vi "CH1_Rx_TCPIP.vi"() -> ()   [LabVIEW 2018]
uses:
  RxTx/RxTx.lvclass
  TCPIP/TCPIP.lvclass
  TCPIP/TCPIP.lvclass/TCPIP.ctl
panel:
  in  "TCPIP.lvclass":refnum<class "TCPIP.lvclass">
  in  "remote port":u16=2000
  in  "IP":string="200.131.64.48"
  in  "RxTx.lvclass":refnum<class "RxTx.lvclass">
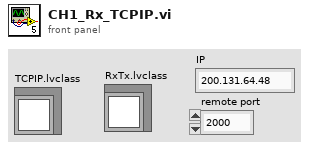
[diagram p1: front panel]
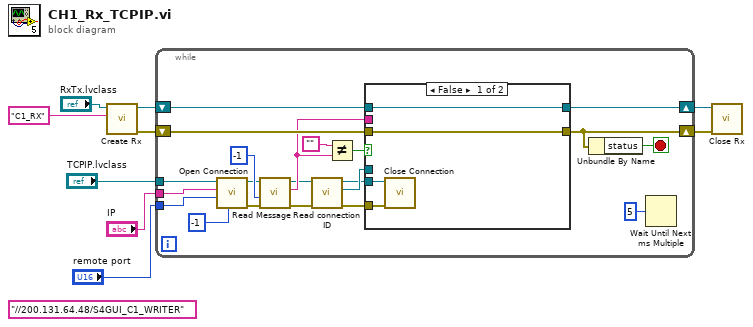
[diagram p0: block diagram]
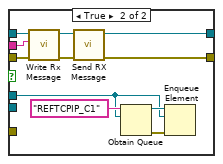
[diagram p2: hidden frame]
diagram:
  (unwired) "//200.131.64.48/S4GUI_C1_WRITER" ("witer name")
  n1 = call "Create Rx.vi"("Reader Name"="C1_RX", "RxTx in"="RxTx.lvclass") -> ("error out"=w6:errorcluster, "RxTx out"=w7:refnum<class "RxTx.lvclass">)  [unwired: 8 in]
  n2 = while {
    shift-right: [w27] -> w4
    shift-left: w6 -> [w30]
    shift-right: [w28] -> w5
    shift-left: w7 -> [w29]
    tunnel: "IP" -> [w23]
    tunnel: "remote port" -> [w22]
    tunnel: "TCPIP.lvclass" -> [w13]
    stop <- w24 stop-if-true
    n3 = call "Open Connection.vi"("timeout"=-1, "remote port"=w22, "IP"=w23, "TCPIP in"=w13) -> ("error out"=w19:errorcluster, "TCPIP out"=w20:refnum<class "TCPIP.lvclass">)  [unwired: 6 in]
    n4 = call "Read Message.vi"("error in (no error)"=w19, "timeout"=-1, "TCPIP in"=w20) -> ("error out"=w17:errorcluster, "Message"=w18:string, "TCPIP out"=w16:refnum<class "TCPIP.lvclass">)  [unwired: 6 in]
    n5 = call "Read connection ID.vi"("error in (no error)"=w17, "TCPIP in"=w16) -> ("error out"=w11:errorcluster, "connection ID"=w15:refnum<k5>, "TCPIP out"=w12:refnum<class "TCPIP.lvclass">)  [unwired: 7 in]
    n6 = Not Equal?(x="", y=w18) -> (x != y?=w25:bool)
    n7 = case shown="False" w25 {
      tunnel: w30 -> [w33 w43]
      tunnel: w29 -> [w34 w42]
      tunnel: [w34 w40] -> w28
      tunnel: [w33 w39] -> w27
      tunnel: w18 -> [_ w41]
      tunnel: w15 -> [_ w35]
      tunnel: w12 -> [w32 _]
      tunnel: w11 -> [w31 _]
      frame False {
        n8 = call "Close Connection.vi"("error in (no error)"=w31, "TCPIP in"=w32) -> ()  [unwired: 8 in, 2 out]
      }
      frame True {
        n9 = call "Write Rx Message.vi"("error in (no error)"=w43, "Rx Message"=w41, "RxTx in"=w42) -> ("error out"=w44:errorcluster, "RxTx out"=w45:refnum<class "RxTx.lvclass">)  [unwired: 7 in]
        n10 = call "Send RX Message.vi"("error in (no error)"=w44, "RxTx in"=w45) -> ("error out"=w39:errorcluster, "RxTx out"=w40:refnum<class "RxTx.lvclass">)  [unwired: 8 in]
        n11 = Obtain Queue(name (unnamed)="REFTCPIP_C1", element data type=w35) -> (queue out=w36:refnum<queue>, error out=w37:errorcluster)  [unwired: 3 in, 1 out]
        n12 = Enqueue Element(queue=w36, element=w35, error in (no error)=w37) -> ()  [unwired: 1 in, 3 out]
      }
    }
    n13 = Unbundle By Name(w27) -> ("status"=w24:bool)
    n14 = Wait Until Next ms Multiple(millisecond multiple=u32 5) -> ()  [unwired: 1 out]
  }
  n15 = call "Close Rx.vi"("error in (no error)"=w4, "RxTx in"=w5) -> ()  [unwired: 8 in, 2 out]
